vi "MasterAquisitionFile_LD_IOS.vi"() -> ()   [LabVIEW 2018]
uses:
  <vilib>/userdefined/High Color/IMAQdx.ctl
  <vilib>/vision/driver/IMAQdx.llb/IMAQdx Camera Control Mode.ctl
  <vilib>/vision/driver/IMAQdx.llb/IMAQdx Acquisition Mode.ctl
  <vilib>/vision/driver/IMAQdx.llb/IMAQdx Buffer Number Mode.ctl
  <vilib>/DAQmx/write.llb/DAQmx Write (Digital Bool 1Line 1Point).vi
  <vilib>/DAQmx/read.llb/DAQmx Read (Analog 1D Wfm NChan NSamp).vi
  <vilib>/DAQmx/write.llb/DAQmx Write (Digital 1D Bool NChan 1Samp 1Line).vi
  <vilib>/DAQmx/create/channels.llb/DAQmx Create Channel (DO-Digital Output).vi
  <vilib>/DAQmx/create/channels.llb/DAQmx Create Channel (CO-Pulse Generation-Frequency).vi
  <vilib>/DAQmx/configure/timing.llb/DAQmx Timing (Implicit).vi
  <vilib>/DAQmx/create/channels.llb/DAQmx Create Channel (AI-Voltage-Basic).vi
  <vilib>/DAQmx/configure/timing.llb/DAQmx Timing (Sample Clock).vi
  <vilib>/DAQmx/configure/trigger.llb/DAQmx Start Trigger (Digital Edge).vi
  <vilib>/DAQmx/miscellaneous.llb/DAQmx Fill In Error Info.vi
  <vilib>/vision/driver/NI_Vision_Acquisition_Software.lvlib
  <resource>/objmgr/imaqdx.rc
panel:
  out "Dev2 Analog Samples":i32
  out "Dev2 Analog":bool
  in  "stop 2":bool
  out "CBV Camera 2":bool
  in  "Dev2 Channels":tag="Dev2/ai4:5"
  in  "Dev2 Analog Channels":string[](array[string])=["LD_BackScatter", "LD_Flow", "LPadSol", "RPadSol", "AudSol", "Hippocampus", "EMG", "Cortical_RH"]
  out "?":T1(plugin-control)
  out "?":T1(plugin-control)
  out "?":T1(plugin-control)
  out "?":T1(plugin-control)
  in  "stop":bool
  out "CBV Cam":bool
  out "Pupil Cam":bool
  out "Whisk Cam":bool
  out "Web Cam":bool
  out "Dev1 Analog":bool
  in  "Dev1 Channels":tag="Dev1/ai0:7"
  out "Web Cam Fs":dbl(knob) scale=0.0..200.0
  out "CBV Cam":dbl(knob) scale=0.0..200.0
  out "Whisk Cam Fs":dbl(knob) scale=0.0..200.0
  out "Last Whisk\nBuffer 2":u32
  out "Pupil Cam Fs":dbl(knob) scale=0.0..200.0
  out "Dropped 2":u32(slide) caption="Pupil Cam" scale=0.0..90.0
  in  "Pupil Cam ID":T2="cam2"
  in  "Pupil Cam Trig Source":tag="Dev2/ctr0"
  in  "Exposure Time (microsec)":string="10000"
  out "Solenoids":bool[](array[boolean])
  out "Dev1 Analog Samples":i32
  in  "Dev1 Analog Channels":string[](array[string])=["Cortical_LH", "Force_Sensor", "LPadSol", "RPadSol", "AudSol", "Hippocampus", "EMG", "Cortical_RH"]
  in  "Whisker Cam ID":T2="cam1"
  in  "WebCam ID":T2="cam0"
  in  "Analog Acquisition":cluster{"Analog Fs":u16}={"Analog Fs"=20000} {"Analog Fs" format="%0.0f"}
  in  "Camera Acquisition Setup":T3={"CBV Cam Fs"=30, "Whisk Cam Fs"=150, "Web Cam Fs"=15, "Pupil Cam Fs"=30}
  out "Notes Size":i32=7
  out "Notes Reversed":string[](array[string])=["Experimenter", "Animal ID", "Hemisphere", "Solenoid PSI", "Isoflurane time", "Session ID", "Amplifier Gain"]
  out "Notes Array":string[](array[string])=["Amplifier Gain", "Session ID", "Isoflurane time", "Solenoid PSI", "Hemisphere", "Animal ID", "Experimenter"]
  in  "Notes:":T4={"Experimenter"="Kevin", "Animal ID"="T109", "Hemisphere"="Both", "Solenoid PSI"="10", "Isoflurane time"="1320", "Session ID"="Imaging Session Seven", "Amplifier Gain"="10000"}
  in  "Whisk Cam Trig Source":tag="Dev1/ctr1"
  in  "CBV Cam Trig Source":tag="Dev1/ctr0"
  in  "Left Pad":tag="Dev1/port0/line0"
  in  "Right Pad":tag="Dev1/port0/line1"
  in  "Auditory":tag="Dev1/port0/line2"
  in  "Offset (s)":dbl=15.0
  in  "Duration (s)":dbl=0.1 step=0.1
  in  "Interval (s)":dbl=30.0
  in  "Right Pad":dbl=1.0
  in  "Left Pad":dbl=1.0
  in  "Auditory":dbl=1.0
  in  "Target Path":path=path "D:/T109/Imaging Session Seven 9.5.19" caption="Final saved file location"
  out "Dropped":u32(slide) caption="Whisk Cam" scale=0.0..450.0
  out "Current file name":string="190905_13_40_55"
  out "CBV Camera":bool
  out "Time Elapsed (Min)":cluster{dbl, dbl}(slide)={15.0, 0.00046676000000000004} scale=0.0..15.0 scale format="%#_2g"
  in  "Time (min)":dbl(knob)=15.0 min=0.5 max=20.0 step=0.5 scale=0.0..20.0 scale format="%#_2g"
  in  "Temp Path":path=path "D:/LabVIEW Streamed Data" caption="Temporary path for streamed data"
  out "Last CBV\nBuffer":i32
  out "Last Whisk\nBuffer":u32=5
  # "Stimuli"
  # "LPAD"
  # "RPAD"
  # "AUD"
  # "Whisk Cam ID"
  # "Pupil Cam ID"
  # "Ratio"
  # "Web Cam ID"
  # "Data Sampling Rates"
  # "Ratio"
  # "Ratio"
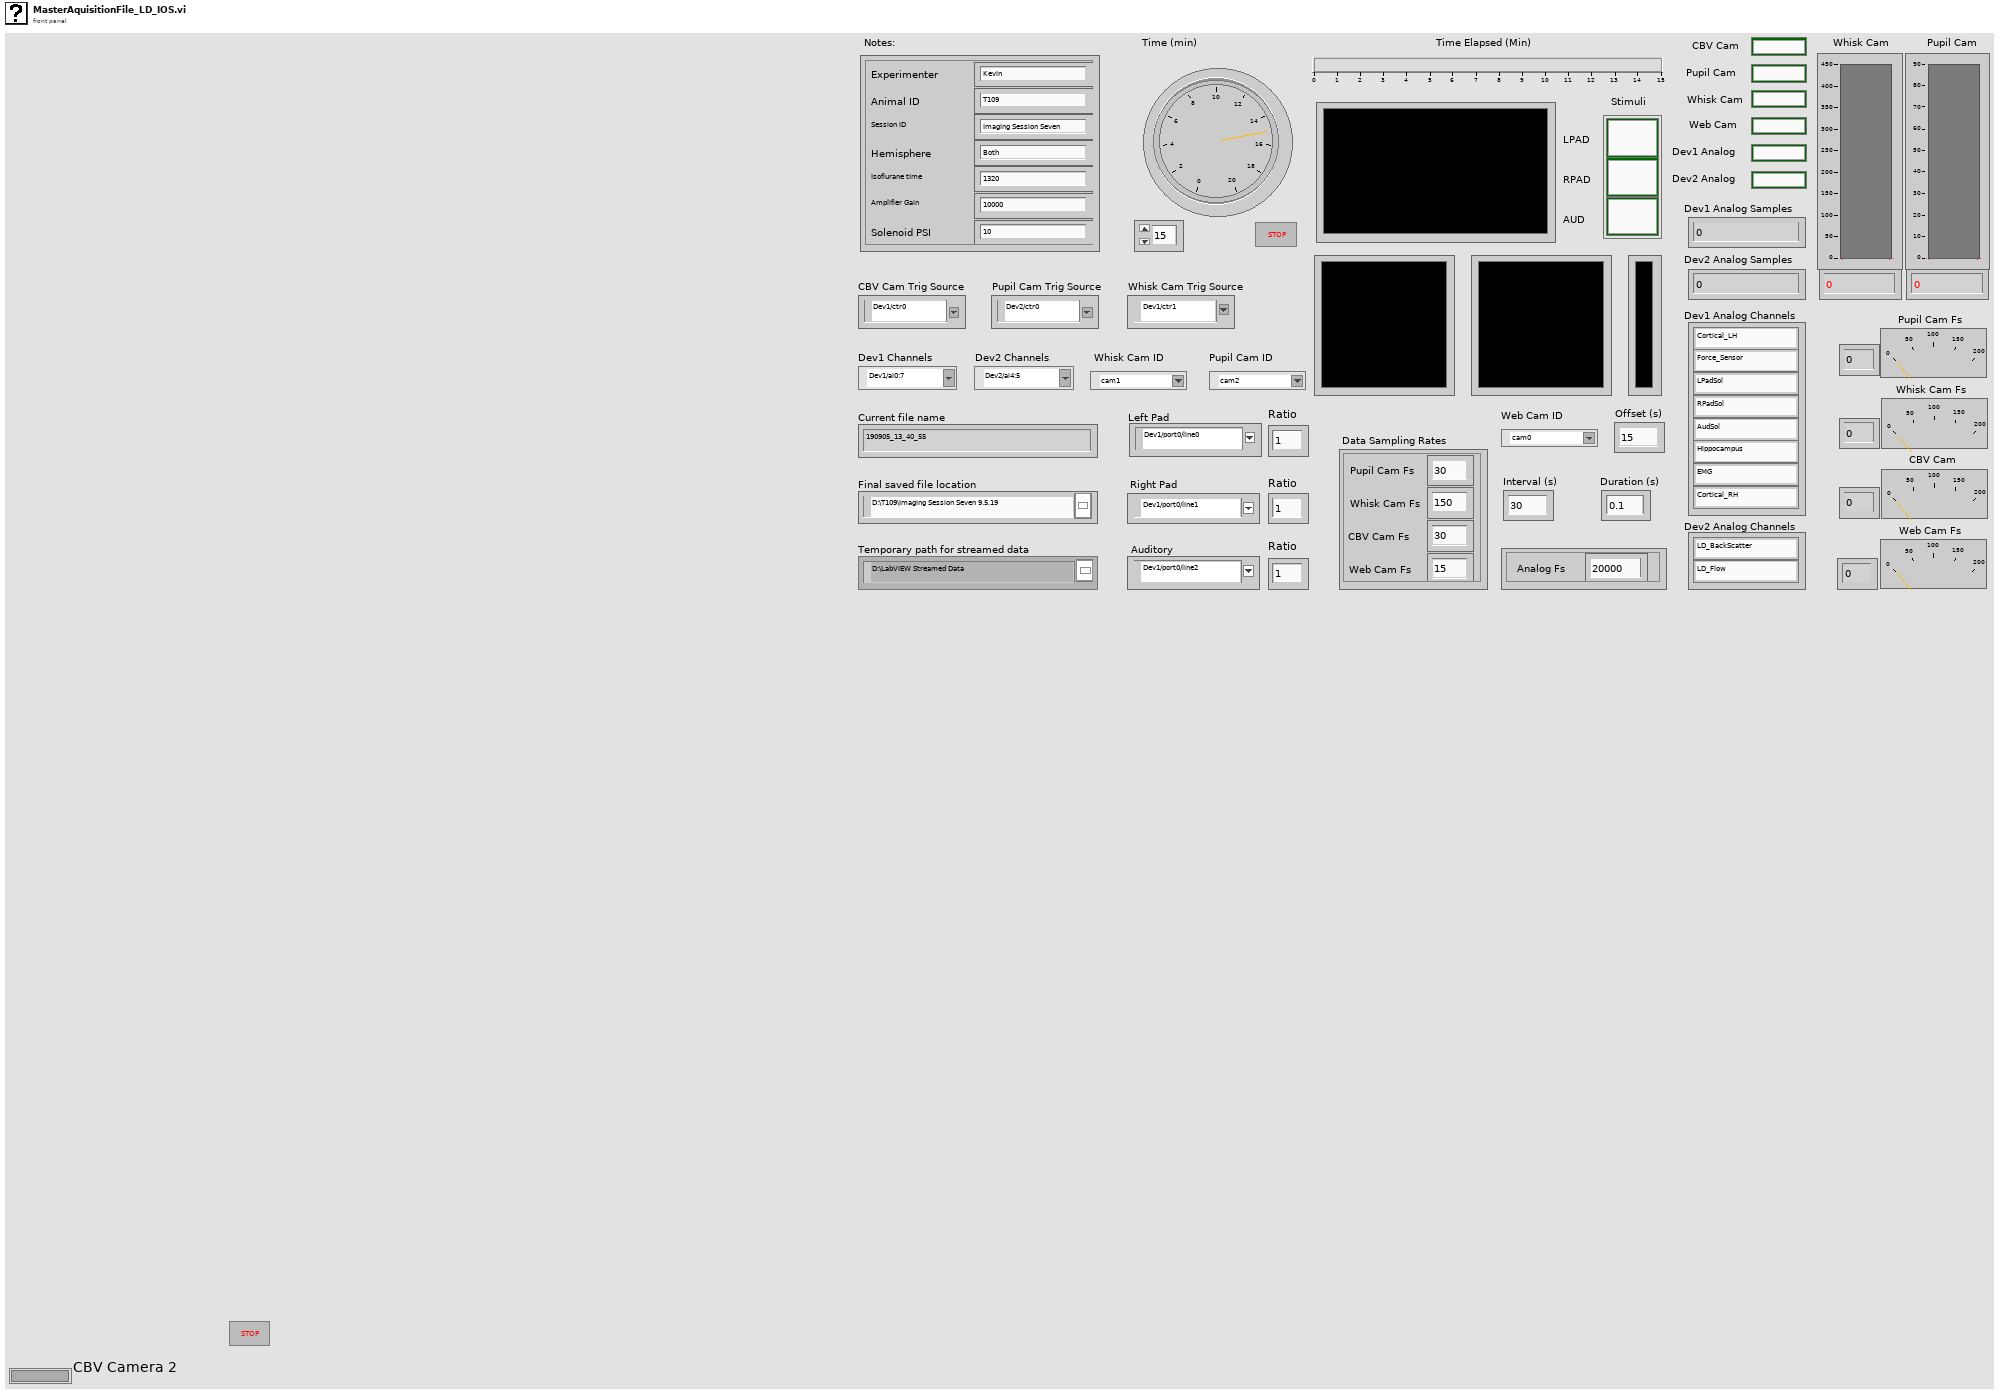
[diagram p1: front panel]
types:
  T1 = typedef "IMAQ Image.ctl" = refnum<image>
  T2 = typedef "IMAQdx.ctl" = refnum<k21>
  T3 = cluster{"CBV Cam Fs":u16, "Whisk Cam Fs":u16, "Web Cam Fs":u16, "Pupil Cam Fs":u16}
  T4 = cluster{"Experimenter":string, "Animal ID":string, "Hemisphere":string, "Solenoid PSI":string, "Isoflurane time":string, "Session ID":string, "Amplifier Gain":string}
  T5 = enum16{"open", "open or create", "create or replace", "create", "open (read-only)"}
  T6 = enum16{"open", "replace", "create", "open or create", "replace or create", "replace or create with confirmation"}
  T7 = typedef "Image Type" = u32
  T8 = typedef "NI_Vision_Acquisition_Software.lvlib/IMAQdx Acquisition Mode.ctl" = enum32{"One Shot", "Continuous"}
  T9 = typedef "NI_Vision_Acquisition_Software.lvlib/IMAQdx Camera Control Mode.ctl" = enum32{"Controller", "Listener"}
  T10 = typedef "IMAQ AVI2 Refnum.ctl" = refnum<k20>
  T11 = enum16{"big-endian, network order", "native, host order", "little-endian"}
  T12 = typedef "NI_Vision_Acquisition_Software.lvlib/IMAQdx Buffer Number Mode.ctl" = enum32{"Next", "Last", "Buffer Number", "Every", "Last New"}
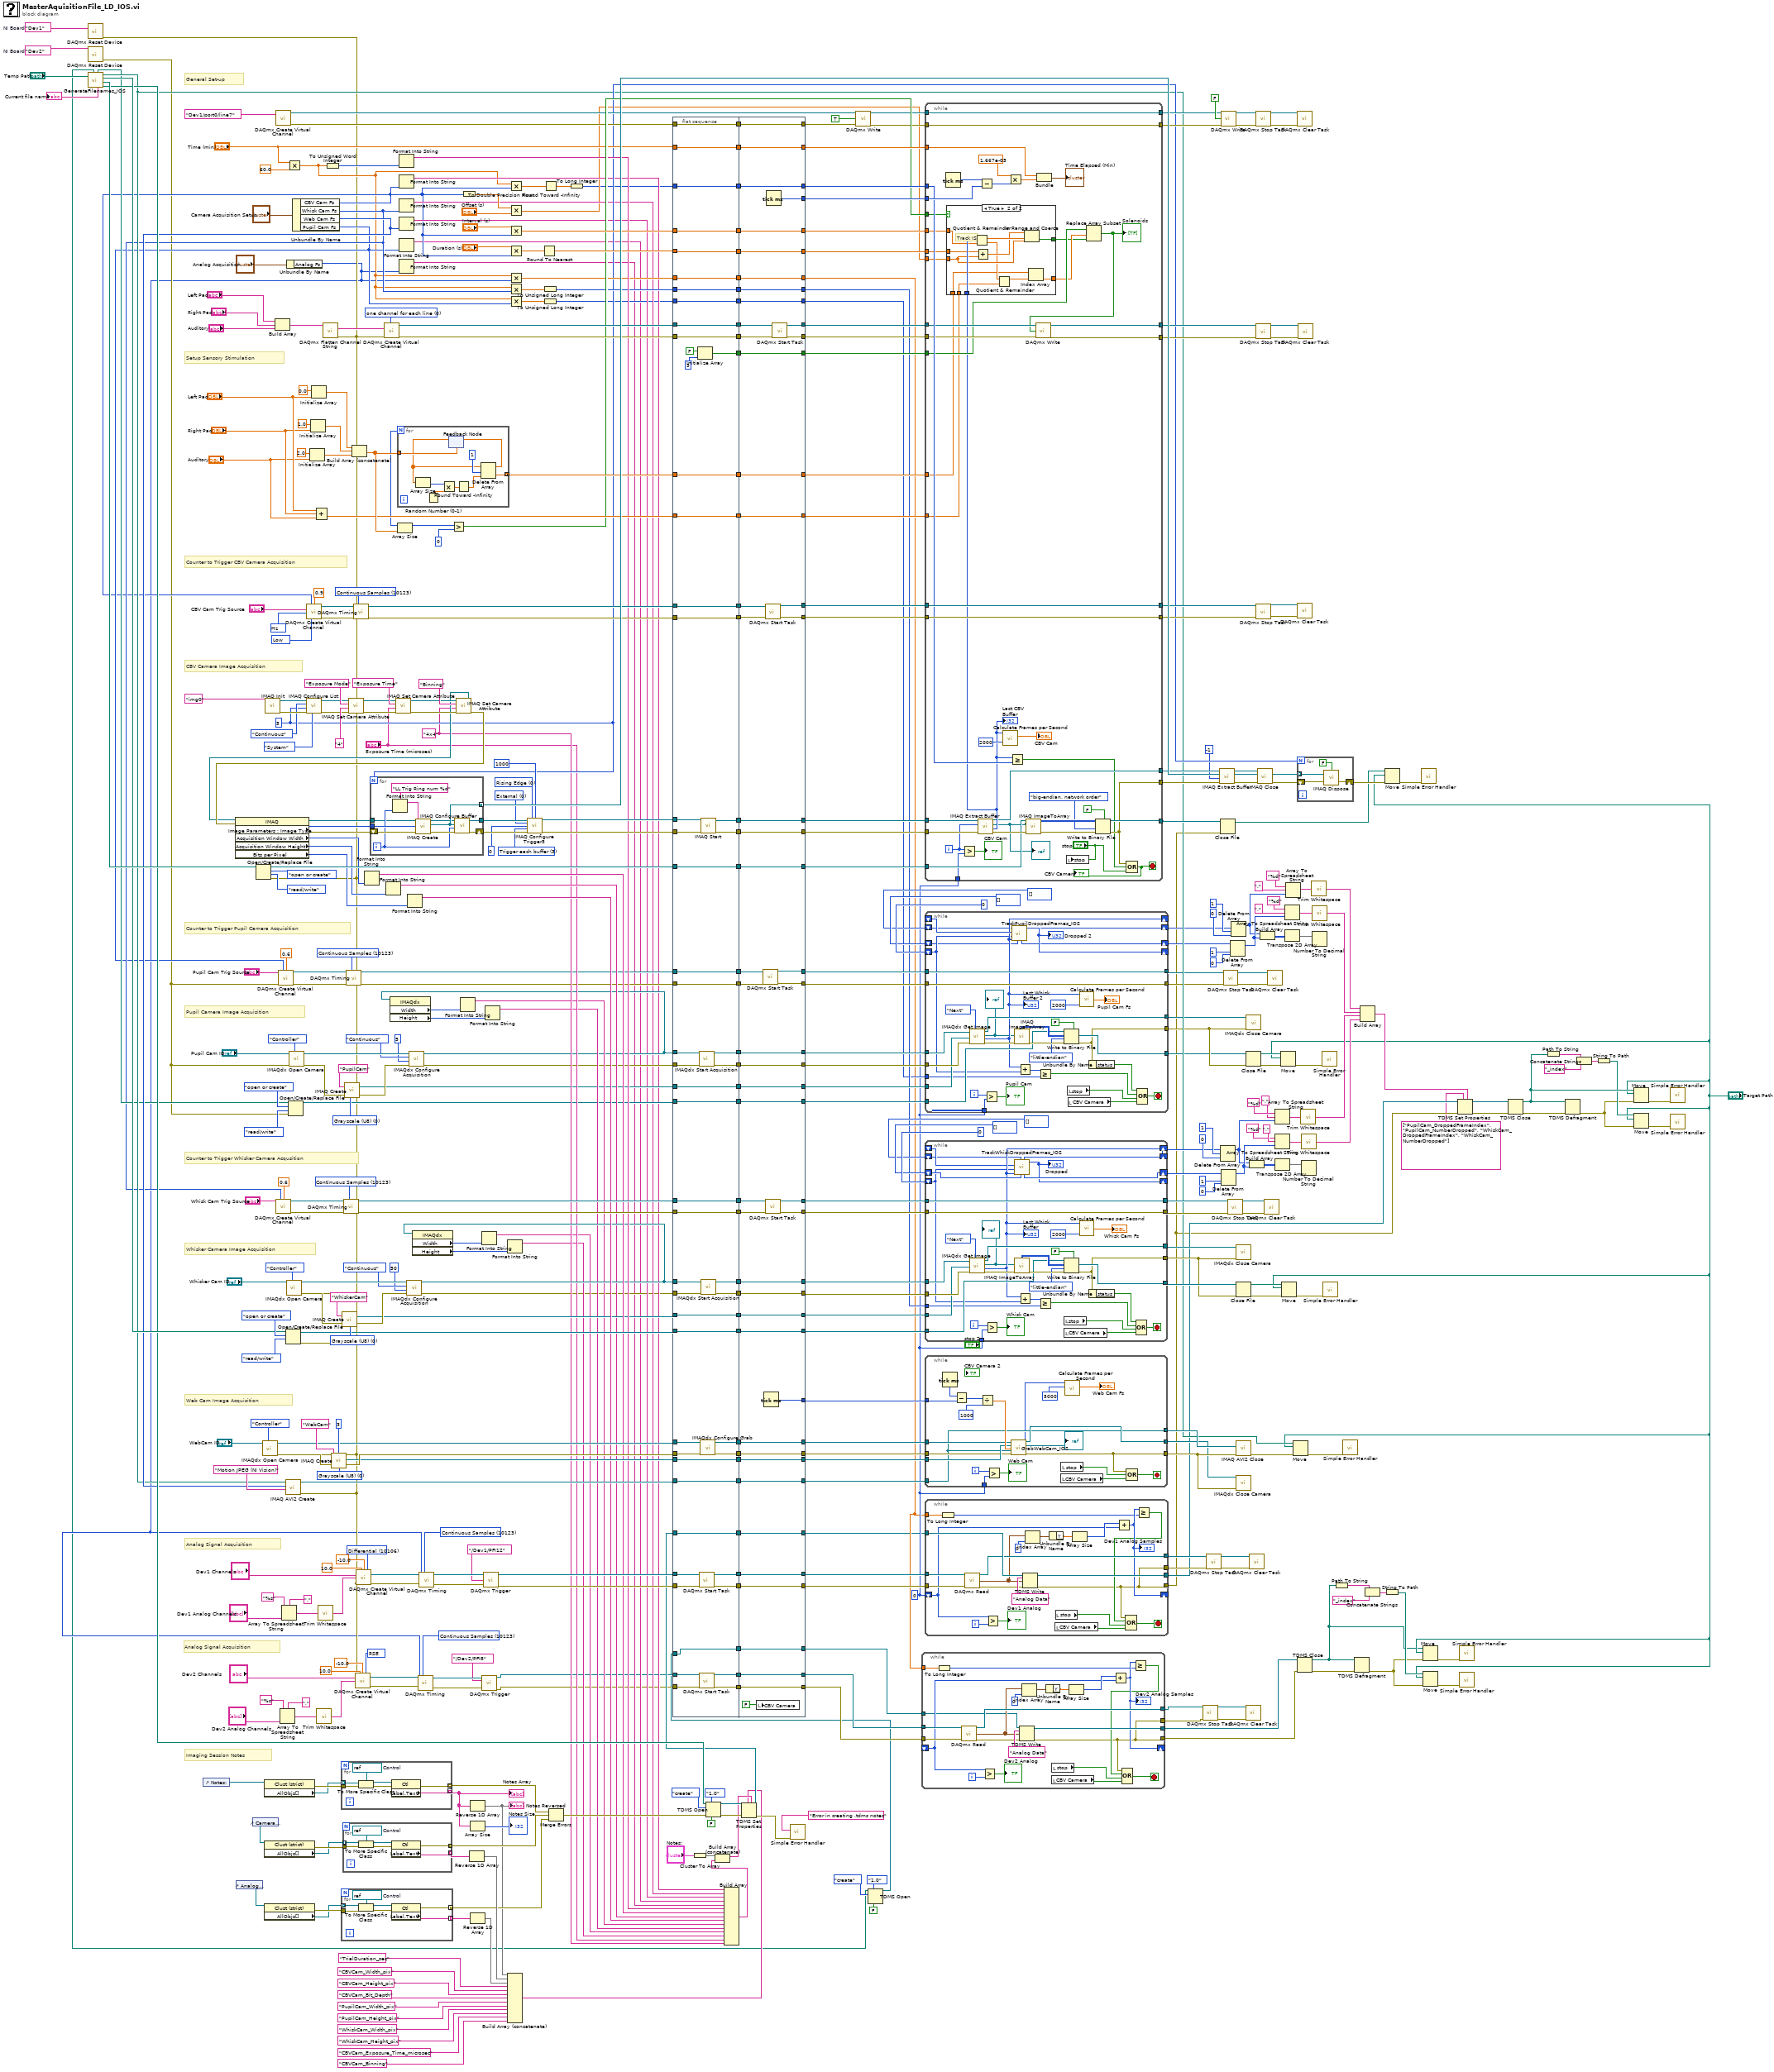
[diagram p0: block diagram]
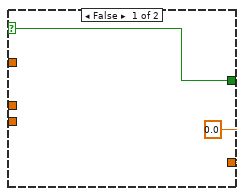
[diagram p2: hidden frame]
diagram:
  w46 = 10123 items=["Finite Samples"=10178, "Continuous Samples"=10123, "Hardware Timed Single Point"=12522] ("sample mode")
  w49 = 10083 items=["default"=-1, "RSE"=10083, "NRSE"=10078, "Differential"=10106, "Pseudodifferential"=12529] ("input terminal configuration")
  w66 = tag "Dev2"  # NI Board
  w153 = 10123 items=["Finite Samples"=10178, "Continuous Samples"=10123, "Hardware Timed Single Point"=12522] ("sample mode")
  w160 = T7 0 items=["Grayscale (U8)", "Grayscale (I16)", "Grayscale (SGL)", "Complex (CSG)", "RGB (U32)", "HSL (U32)", "RGB (U64)", "Grayscale (U16)"] ("Image Type")
  w142 = "4x4" ("Attribute Value")
  w72 = 0
  w326 = 0 items=["one channel for each line", "one channel for all lines"] ("line grouping")
  w377 = 10123 items=["Finite Samples"=10178, "Continuous Samples"=10123, "Hardware Timed Single Point"=12522] ("sample mode")
  w380 = 10106 items=["default"=-1, "RSE"=10083, "NRSE"=10078, "Differential"=10106, "Pseudodifferential"=12529] ("input terminal configuration")
  w431 = T7 0 items=["Grayscale (U8)", "Grayscale (I16)", "Grayscale (SGL)", "Complex (CSG)", "RGB (U32)", "HSL (U32)", "RGB (U64)", "Grayscale (U16)"] ("Image Type")
  w451 = u32 0 items=["Rising Edge", "Falling Edge"] ("Trigger Polarity")
  w454 = u32 0 items=["External"=0, "RTSI"=1, "ISO In"=2, "Scaled Encoder"=5] ("Trigger Type")
  w445 = tag "Dev1"  # NI Board
  w446 = 10123 items=["Finite Samples"=10178, "Continuous Samples"=10123, "Hardware Timed Single Point"=12522] ("sample mode")
  w449 = 10373 items=["Hz"=10373] ("units")
  w450 = 10214 items=["High"=10192, "Low"=10214] ("idle state")
  w172 = u32 5 ("Number of Buffers")
  w452 = u32 3 items=["Disabled", "Trigger start of acquisition", "Trigger start of each buffer list", "Trigger each buffer", "Trigger each line (linescan)", "Trigger end of acquisition"] ("Action")
  w466 = 10123 items=["Finite Samples"=10178, "Continuous Samples"=10123, "Hardware Timed Single Point"=12522] ("sample mode")
  w473 = T7 0 items=["Grayscale (U8)", "Grayscale (I16)", "Grayscale (SGL)", "Complex (CSG)", "RGB (U32)", "HSL (U32)", "RGB (U64)", "Grayscale (U16)"] ("Image Type")
  # "Analog Signal Acquisition"
  # "General Set-up"
  # "Pupil Camera Image Acquisition"
  # "Counter to Trigger Pupil Camera Acquisition"
  # "Whisker Camera Image Acquisition"
  # "Imaging Session Notes"
  # "Setup Sensory Stimulation"
  # "CBV Camera Image Acquisition"
  # "Counter to Trigger CBV Camera Acquisition"
  # "Counter to Trigger Whisker Camera Acqusition"
  # "Web Cam Image Acquisition"
  # "Analog Signal Acquisition"
  n1 = call <vilib>:"DAQmx Reset Device.vi"("device in"=w445) -> ("error out"=w35:errorcluster)  [unwired: 14 in]
  n2 = call <vilib>:"DAQmx Reset Device.vi"("device in"=w66) -> ("error out"=w65:errorcluster)  [unwired: 14 in]
  n3 = call "GenerateFilenames_IOS.vi"("path"="Temp Path") -> ("TDMS Path"=w282:path, "Dalsa Path"=w438:path, "Basler Path"=w434:path, "WebCam Path"=w171:path, "Analog file name"=→"Current file name":string, "Basler2 Path"=w151:path, "TDMS Path 2"=w2:path)  [unwired: 3 in, 1 out]
  n4 = control-ref of="Notes:"() -> (w287:refnum<vi>)
  n5 = control-ref of="Analog Acquisition"() -> (w265:refnum<vi>)
  n6 = control-ref of="Camera Acquisition Setup"() -> (w266:refnum<vi>)
  n7 = Open/Create/Replace File(file path (use dialog)=w438, error in=w35, operation (0:open)=T6."open or create", access (0:read/write)=enum16{"read/write", "read-only", "write-only"}."read/write") -> (refnum out=w381:refnum<file>)  [unwired: 2 in, 2 out]
  n8 = call <vilib>:"IMAQdx Open Camera.vi"("Camera Control Mode"=IMAQdx_Camera_Control_Mode."Controller", "error in"=w35, "Session In"="WebCam ID") -> ("error out"=w427:errorcluster, "Session Out"=w425:T2)  [unwired: 7 in]
  n9 = property class="Clust (strict)"(reference=w287) -> (error out=w290:errorcluster, "AllObjs[]"=w179:refnum<vi>[])  [unwired: 1 in, 1 out]
  n10 = property class="Clust (strict)"(reference=w266) -> (error out=w285:errorcluster, "AllObjs[]"=w180:refnum<vi>[])  [unwired: 1 in, 1 out]
  n11 = property class="Clust (strict)"(reference=w265) -> (error out=w264:errorcluster, "AllObjs[]"=w178:refnum<vi>[])  [unwired: 1 in, 1 out]
  n12 = call <vilib>:"IMAQ Init.vi"("error in (no error)"=w35, "Interface Name"="img0") -> ("error out"=w464:errorcluster, "IMAQ Session Out"=w465:refnum<k11>)  [unwired: 8 out]
  n13 = Build Array("Left Pad", "Right Pad", "Auditory") -> (w58:tag[])
  n14 = call-poly <vilib>:"DAQmx Create Virtual Channel.vi"("lines"=tag "Dev1/port0/line7") -> ("task out"=w212:refnum<k21>, "error out"=w215:errorcluster)  [unwired: 13 in]
  n15 = Array To Spreadsheet String(delimiter (Tab)=",", array="Dev2 Analog Channels", 3:"%s" ("format string")) -> (spreadsheet string=w39:string)
  n16 = Array To Spreadsheet String(delimiter (Tab)=",", array="Dev1 Analog Channels", 3:"%s" ("format string")) -> (spreadsheet string=w251:string)
  n17 = Open/Create/Replace File(file path (use dialog)=w434, error in=w35, operation (0:open)=T6."open or create", access (0:read/write)=enum16{"read/write", "read-only", "write-only"}."read/write") -> (refnum out=w399:refnum<file>)  [unwired: 2 in, 2 out]
  n18 = Unbundle By Name("Analog Acquisition") -> ("Analog Fs"=w34:u16)
  n19 = call <vilib>:"IMAQdx Open Camera.vi"("Camera Control Mode"=IMAQdx_Camera_Control_Mode."Controller", "error in"=w35, "Session In"="Whisker Cam ID") -> ("error out"=w476:errorcluster, "Session Out"=w479:T2)  [unwired: 7 in]
  n20 = Multiply(x="Time (min)", y=60.0) -> (x*y=w74:dbl)
  n21 = Open/Create/Replace File(file path (use dialog)=w151, error in=w65, operation (0:open)=T6."open or create", access (0:read/write)=enum16{"read/write", "read-only", "write-only"}."read/write") -> (refnum out=w132:refnum<file>)  [unwired: 2 in, 2 out]
  n22 = call <vilib>:"IMAQdx Open Camera.vi"("Camera Control Mode"=IMAQdx_Camera_Control_Mode."Controller", "error in"=w65, "Session In"="Pupil Cam ID") -> ("error out"=w163:errorcluster, "Session Out"=w166:T2)  [unwired: 7 in]
  n23 = Unbundle By Name("Camera Acquisition Setup") -> ("CBV Cam Fs"=w76:u16, "Whisk Cam Fs"=w114:u16, "Web Cam Fs"=w259:u16, "Pupil Cam Fs"=w108:u16)
  n24 = call-poly <vilib>:"DAQmx Create Virtual Channel.vi"("frequency"=w114, "duty cycle"=0.6, "counter"="Whisk Cam Trig Source", "error in"=w35) -> ("task out"=w468:refnum<k21>, "error out"=w467:errorcluster)  [unwired: 10 in]
  n25 = call-poly <vilib>:"DAQmx Create Virtual Channel.vi"("frequency"=w108, "duty cycle"=0.6, "counter"="Pupil Cam Trig Source", "error in"=w65) -> ("task out"=w155:refnum<k21>, "error out"=w154:errorcluster)  [unwired: 10 in]
  n26 = call "IMAQ AVI2 Create"("error in (no error)"=w35, "Codec"="Motion JPEG (NI Vision)", "Frames Per Second"=w259, "AVI Path"=w171) -> ("AVI Refnum"=w417:T10)  [unwired: 6 in, 1 out]
  n27 = call <vilib>:"IMAQ Configure List.vi"("Memory Location"=enum16{"System", "Onboard"}."System", "error in (no error)"=w464, "Number of buffers"=w172, "Continuous?"=enum16{"One-Shot", "Continuous"}."Continuous" ("Continuous ?"), "IMAQ Session In"=w465) -> ("error out"=w193:errorcluster, "IMAQ Session Out"=w189:refnum<k11>)  [unwired: 1 in, 4 out]
  n28 = call-poly <vilib>:"DAQmx Create Virtual Channel.vi"("frequency"=w76, "duty cycle"=0.9, "counter"="CBV Cam Trig Source", "units"=w449, "error in"=w35, "idle state"=w450) -> ("task out"=w448:refnum<k21>, "error out"=w447:errorcluster)  [unwired: 8 in]
  n29 = Initialize Array(2.0 ("element"), "Auditory") -> (w70:dbl[])
  n30 = Initialize Array(1.0 ("element"), "Right Pad") -> (w330:dbl[])
  n31 = Initialize Array(0.0 ("element"), "Left Pad") -> (w331:dbl[])
  n32 = Compound Arithmetic op=ADD("Left Pad", "Right Pad", "Auditory") -> (w310:dbl)
  n33 = call <vilib>:"Trim Whitespace.vi"("string"=w39) -> ("trimmed string"=w38:string)  [unwired: 1 in]
  n34 = call <vilib>:"Trim Whitespace.vi"("string"=w251) -> ("trimmed string"=w250:string)  [unwired: 1 in]
  n35 = call <vilib>:"DAQmx Flatten Channel String.vi"("names in"=w58, "error in"=w35) -> ("names out"=w292:string, "error out"=w291:errorcluster)  [unwired: 12 in]
  n36 = To Unsigned Word Integer(number=w74) -> (unsigned 16bit integer=w245:u16)
  n37 = call "IMAQ Create"("Border Size"=3, "Image Name"="WebCam", "Image Type"=w431, "error in (no error)"=w427) -> ("New Image"=w424:T1, "error out"=w426:errorcluster)  [unwired: 1 in]
  n38 = for {
    tunnel: [w485] -> w289 mode=indexing
    tunnel: w290 -> [w484]
    tunnel: [w482] -> w273 mode=indexing
    tunnel: w179 -> [w481] mode=indexing
    w486 = refnum<vi> refnum  # Control
    n39 = To More Specific Class(target class=w486, reference=w481, error in=w484) -> (specific class reference=w487:refnum<vi>, error out=w483:errorcluster)
    n40 = property class="Ctl"(reference=w487, error in=w483) -> (error out=w482:errorcluster, "Label.Text"=w485:string)  [unwired: 1 out]
  }
  "Notes Array" <- w289
  n41 = for {
    tunnel: [w492] -> w262 mode=indexing
    tunnel: w264 -> [w491]
    tunnel: [w489] -> w263 mode=indexing
    tunnel: w178 -> [w488] mode=indexing
    w493 = refnum<vi> refnum  # Control
    n42 = To More Specific Class(target class=w493, reference=w488, error in=w491) -> (specific class reference=w494:refnum<vi>, error out=w490:errorcluster)
    n43 = property class="Ctl"(reference=w494, error in=w490) -> (error out=w489:errorcluster, "Label.Text"=w492:string)  [unwired: 1 out]
  }
  n44 = call "IMAQ Create"("Image Name"="WhiskerCam", "Image Type"=w473, "error in (no error)"=w476) -> ("New Image"=w232:T1, "error out"=w474:errorcluster)  [unwired: 2 in]
  n45 = for {
    tunnel: [w499] -> w286 mode=indexing
    tunnel: w285 -> [w498]
    tunnel: [w496] -> w272 mode=indexing
    tunnel: w180 -> [w495] mode=indexing
    w500 = refnum<vi> refnum  # Control
    n46 = To More Specific Class(target class=w500, reference=w495, error in=w498) -> (specific class reference=w501:refnum<vi>, error out=w497:errorcluster)
    n47 = property class="Ctl"(reference=w501, error in=w497) -> (error out=w496:errorcluster, "Label.Text"=w499:string)  [unwired: 1 out]
  }
  n48 = call-poly <vilib>:"DAQmx Timing.vi"("task/channels in"=w468, "sample mode"=w466, "error in"=w467) -> ("task out"=w362:refnum<k21>, "error out"=w360:errorcluster)  [unwired: 11 in]
  n49 = call "IMAQ Create"("Image Name"="PupilCam", "Image Type"=w160, "error in (no error)"=w163) -> ("New Image"=w117:T1, "error out"=w161:errorcluster)  [unwired: 2 in]
  n50 = call-poly <vilib>:"DAQmx Timing.vi"("task/channels in"=w155, "sample mode"=w153, "error in"=w154) -> ("task out"=w130:refnum<k21>, "error out"=w128:errorcluster)  [unwired: 11 in]
  n51 = call <vilib>:"IMAQ Set Camera Attribute.vi"("error in (no error)"=w193, "Attribute Value"="4", "Camera Attribute"="Exposure Mode", "IMAQ Session In"=w189) -> ("error out"=w192:errorcluster, "IMAQ Session Out"=w188:refnum<k11>)  [unwired: 4 in]
  n52 = Build Array (concatenate)(w331, w330, w70) -> (w329:dbl[])
  n53 = call-poly <vilib>:"DAQmx Timing.vi"("task/channels in"=w448, "sample mode"=w446, "error in"=w447) -> ("task out"=w366:refnum<k21>, "error out"=w364:errorcluster)  [unwired: 11 in]
  n54 = call-poly <vilib>:"DAQmx Create Virtual Channel.vi"("maximum value"=10.0, "minimum value"=-10.0, "input terminal configuration"=w49, "physical channels"="Dev2 Channels", "name to assign"=w38, "error in"=w35) -> ("task out"=w48:refnum<k21>, "error out"=w47:errorcluster)  [unwired: 8 in]
  n55 = call-poly <vilib>:"DAQmx Create Virtual Channel.vi"("maximum value"=10.0, "minimum value"=-10.0, "input terminal configuration"=w380, "physical channels"="Dev1 Channels", "name to assign"=w250, "error in"=w35) -> ("task out"=w379:refnum<k21>, "error out"=w378:errorcluster)  [unwired: 8 in]
  n56 = call-poly <vilib>:"DAQmx Create Virtual Channel.vi"("lines"=w292, "line grouping"=w326, "error in"=w291) -> ("task out"=w324:refnum<k21>, "error out"=w322:errorcluster)  [unwired: 11 in]
  n57 = call <vilib>:"IMAQ Set Camera Attribute.vi"("error in (no error)"=w192, "Attribute Value"="Exposure Time (microsec)", "Camera Attribute"="Exposure Time", "IMAQ Session In"=w188) -> ("error out"=w191:errorcluster, "IMAQ Session Out"=w187:refnum<k11>)  [unwired: 4 in]
  n58 = Array Size(array=w329) -> (size(s)=w256:i32)
  n59 = for {
    N: w256 -> [_]
    tunnel: w329 -> [w505]
    tunnel: [w502] -> w307 mode=concatenating
    n60 = Random Number (0-1)() -> (number: 0 to 1=w509:dbl)
    n61 = feedback #1(w505) -> (w504:dbl[])
    n62 = Array Size(array=w504) -> (size(s)=w510:i32)
    n63 = Multiply(x=w510, y=w509) -> (x*y=w508:dbl)
    n64 = Round Toward -Infinity(1:w508) -> (0:w507:dbl)
    n65 = Delete From Array(array=w504, length=1, index=w507) -> (deleted portion=w502:dbl[], array with subset deleted=w503:dbl[])
    n66 = feedback-in #1(w503) -> ()
  }
  n67 = Format Into String(w245) -> (resulting string=w247:string)  [unwired: 3 in, 1 out]
  n68 = Format Into String(w76) -> (resulting string=w112:string)  [unwired: 3 in, 1 out]
  n69 = Format Into String(w114) -> (resulting string=w111:string)  [unwired: 3 in, 1 out]
  n70 = Format Into String(w259) -> (resulting string=w110:string)  [unwired: 3 in, 1 out]
  n71 = Format Into String(w108) -> (resulting string=w51:string)  [unwired: 3 in, 1 out]
  n72 = Format Into String(w34) -> (resulting string=w50:string)  [unwired: 3 in, 1 out]
  n73 = call <vilib>:"IMAQdx Configure Acquisition.vi"("error in"=w474, "Number of Buffers"=u32 50, "Continuous?"=IMAQdx_Acquisition_Mode."Continuous", "Session In"=w479) -> ("error out"=w73:errorcluster, "Session Out"=w233:T2)  [unwired: 6 in]
  n74 = call <vilib>:"IMAQdx Configure Acquisition.vi"("error in"=w161, "Number of Buffers"=u32 5, "Continuous?"=IMAQdx_Acquisition_Mode."Continuous", "Session In"=w166) -> ("error out"=w134:errorcluster, "Session Out"=w118:T2)  [unwired: 6 in]
  n75 = property class="IMAQdx"(reference=w118) -> ("Width"=w150:u32, "Height"=w149:u32)  [unwired: 1 in, 2 out]
  n76 = property class="IMAQdx"(reference=w233) -> ("Width"=w244:u32, "Height"=w243:u32)  [unwired: 1 in, 2 out]
  n77 = call-poly <vilib>:"DAQmx Timing.vi"("task/channels in"=w48, "sample mode"=w46, "rate"=w34, "error in"=w47) -> ("task out"=w36:refnum<k21>, "error out"=w45:errorcluster)  [unwired: 10 in]
  n78 = call-poly <vilib>:"DAQmx Timing.vi"("task/channels in"=w379, "sample mode"=w377, "rate"=w34, "error in"=w378) -> ("task out"=w176:refnum<k21>, "error out"=w376:errorcluster)  [unwired: 10 in]
  n79 = Greater?(x=w256, y=0) -> (0:w254:bool)
  n80 = call <vilib>:"IMAQ Set Camera Attribute.vi"("error in (no error)"=w191, "Attribute Value"=w142, "Camera Attribute"="Binning", "IMAQ Session In"=w187) -> ("error out"=w190:errorcluster, "IMAQ Session Out"=w186:refnum<k11>)  [unwired: 4 in]
  n81 = property class="IMAQ"(reference=w186, error in=w190) -> (reference out=w200:refnum<k11>, error out=w199:errorcluster, "Image Parameters : Image Type"=w460:u32, "Acquisition Window Width"=w242:u32, "Acquisition Window Height"=w241:u32, "Bits per Pixel"=w240:u32)
  n82 = Format Into String(w242) -> (resulting string=w239:string)  [unwired: 3 in, 1 out]
  n83 = for {
    N: w172 -> [_]
    tunnel: [w520] -> w456
    tunnel: w460 -> [w518]
    shift-right: [w519] -> w455
    shift-left: w199 -> [w517]
    tunnel: [w512] -> w457 mode=indexing
    tunnel: w200 -> [w511]
    i -> [w513]
    n84 = Format Into String(format string="LL Trig Ring num %d", w513) -> (resulting string=w515:string)  [unwired: 2 in, 1 out]
    n85 = call "IMAQ Create"("Image Name"=w515, "Image Type"=w518, "error in (no error)"=w517) -> ("New Image"=w512:T1, "error out"=w516:errorcluster)  [unwired: 1 in, 1 out]
    n86 = call <vilib>:"IMAQ Configure Buffer.vi"("error in (no error)"=w516, "Buffer Number"=w513, "Image In"=w512, "IMAQ Session In"=w511) -> ("error out"=w519:errorcluster, "IMAQ Session Out"=w520:refnum<k11>)  [unwired: 2 in, 4 out]
  }
  n87 = Format Into String(w241) -> (resulting string=w173:string)  [unwired: 3 in, 1 out]
  n88 = Format Into String(w240) -> (resulting string=w238:string)  [unwired: 3 in, 1 out]
  n89 = Format Into String(w150) -> (resulting string=w137:string)  [unwired: 3 in, 1 out]
  n90 = To Double Precision Float(number=w76) -> (double precision float=w293:dbl)
  n91 = Reverse 1D Array(array=w286) -> (reversed array=w276:string[])
  n92 = Reverse 1D Array(array=w289) -> (reversed array=w177:string[])
  "Notes Reversed" <- w177
  n93 = Array Size(array=w289) -> (size(s)=→"Notes Size":i32)
  n94 = Reverse 1D Array(array=w262) -> (reversed array=w261:string[])
  n95 = Format Into String(w244) -> (resulting string=w139:string)  [unwired: 3 in, 1 out]
  n96 = call-poly <vilib>:"DAQmx Trigger.vi"("task/channels in"=w36, "source"=tag "/Dev2/PFI8", "error in"=w45) -> ("task out"=w33:refnum<k21>, "error out"=w32:errorcluster)  [unwired: 11 in]
  n97 = call-poly <vilib>:"DAQmx Trigger.vi"("task/channels in"=w176, "source"=tag "/Dev1/PFI12", "error in"=w376) -> ("task out"=w375:refnum<k21>, "error out"=w374:errorcluster)  [unwired: 11 in]
  n98 = Format Into String(w149) -> (resulting string=w138:string)  [unwired: 3 in, 1 out]
  n99 = Build Array (concatenate)(w177, w276, w261, "TrialDuration_sec", "CBVCam_Width_pix", "CBVCam_Height_pix", "CBVCam_Bit_Depth", "PupilCam_Width_pix", "PupilCam_Height_pix", "WhiskCam_Width_pix", "WhiskCam_Height_pix", "CBVCam_Exposure_Time_microsec" ("element"), "CBVCam_Binning" ("element")) -> (w168:string[])
  n100 = Format Into String(w243) -> (resulting string=w140:string)  [unwired: 3 in, 1 out]
  n101 = Multiply(x=w74, y=w76) -> (x*y=w436:dbl)
  n102 = Multiply(x="Offset (s)", y=w293) -> (x*y=w106:dbl)
  n103 = Multiply(x="Interval (s)", y=w76) -> (x*y=w314:dbl)
  n104 = Multiply(x="Duration (s)", y=w76) -> (x*y=w301:dbl)
  n105 = Multiply(x=w74, y=w34) -> (x*y=w221:dbl)
  n106 = Multiply(x=w114, y=w74) -> (x*y=w174:dbl)
  n107 = Multiply(x=w108, y=w74) -> (x*y=w113:dbl)
  n108 = call <vilib>:"IMAQ Configure Trigger3.vi"("IMAQ Session In"=w456, "Polarity"=w451, "Frame timeout (ms)"=u32 1000 ("Frame Timeout (ms)"), "Type"=w454, "Line Number"=u32 0 ("Trigger Line Number"), "Action"=w452, "error in (no error)"=w455) -> ("IMAQ Session Out"=w398:refnum<k11>, "error out"=w397:errorcluster)  [unwired: 2 in, 5 out]
  n109 = Round To Nearest(number=w301) -> (nearest integer value=w300:dbl)
  n110 = To Unsigned Long Integer(number=w174) -> (unsigned 32bit integer=w219:u32)
  n111 = To Unsigned Long Integer(number=w113) -> (unsigned 32bit integer=w109:u32)
  n112 = Round Toward -Infinity(1:w436) -> (0:w435:dbl)
  n113 = Merge Errors(w273, w272, w263) -> (w271:errorcluster)
  n114 = To Long Integer(number=w435) -> (32bit integer=w75:i32)
  n115 = flat-sequence {
    tunnel: w426 -> [w574]
    tunnel: w425 -> [w573]
    tunnel: w424 -> [w572]
    tunnel: [w572] -> w423
    tunnel: [w571] -> w421
    tunnel: [w570] -> w419
    tunnel: w417 -> [w569]
    tunnel: [w569] -> w416
    tunnel: w233 -> [w568]
    tunnel: w73 -> [w567]
    tunnel: [w566] -> w406
    tunnel: [w565] -> w404
    tunnel: [w564] -> w402
    tunnel: w232 -> [w564]
    tunnel: [w563] -> w400
    tunnel: w399 -> [w563]
    tunnel: w398 -> [w562]
    tunnel: w397 -> [w561]
    tunnel: [w560] -> w395
    tunnel: [w559] -> w393
    tunnel: w75 -> [w558]
    tunnel: [w558] -> w387
    tunnel: "Time (min)" -> [w557]
    tunnel: [w557] -> w384
    tunnel: [w556] -> w382
    tunnel: w381 -> [w556]
    tunnel: w375 -> [w555]
    tunnel: w374 -> [w554]
    tunnel: [w553] -> w373
    tunnel: [w552] -> w372
    tunnel: [w551] -> w368
    tunnel: w274 -> [w551]
    tunnel: w366 -> [w550]
    tunnel: [w550] -> w365
    tunnel: w364 -> [w549]
    tunnel: [w549] -> w363
    tunnel: w362 -> [w548]
    tunnel: [w548] -> w361
    tunnel: w360 -> [w547]
    tunnel: [w547] -> w359
    tunnel: w324 -> [w546]
    tunnel: [w546] -> w325
    tunnel: w322 -> [w545]
    tunnel: [w545] -> w323
    tunnel: w314 -> [w544]
    tunnel: [w544] -> w313
    tunnel: [w543] -> w311
    tunnel: w300 -> [w543]
    tunnel: w310 -> [w542]
    tunnel: [w542] -> w309
    tunnel: w307 -> [w541]
    tunnel: [w541] -> w306
    tunnel: [w539] -> w304
    tunnel: w221 -> [w537]
    tunnel: [w537] -> w220
    tunnel: w219 -> [w536]
    tunnel: [w536] -> w218
    tunnel: w215 -> [w535]
    tunnel: [w535] -> w214
    tunnel: [w528] -> w136
    tunnel: w118 -> [w529]
    tunnel: [w526] -> w135
    tunnel: w134 -> [w527]
    tunnel: [w534] -> w133
    tunnel: w132 -> [w534]
    tunnel: [w533] -> w131
    tunnel: w130 -> [w533]
    tunnel: [w532] -> w129
    tunnel: w128 -> [w532]
    tunnel: w117 -> [w531]
    tunnel: [w531] -> w116
    tunnel: w109 -> [w530]
    tunnel: [w530] -> w107
    tunnel: w33 -> [w525]
    tunnel: w32 -> [w524]
    tunnel: [w523] -> w31
    tunnel: [w522] -> w30
    tunnel: w5 -> [w521]
    tunnel: [w521] -> w4
    tunnel: [w625] -> w428
    tunnel: w423 -> [w624]
    tunnel: [w624] -> w422
    tunnel: w421 -> [w623]
    tunnel: [w623] -> w420
    tunnel: w419 -> [w622]
    tunnel: [w622] -> w418
    tunnel: w416 -> [w621]
    tunnel: [w621] -> w415
    tunnel: [w603] -> w412
    tunnel: [w602] -> w410
    tunnel: [w620] -> w407
    tunnel: w406 -> [w620]
    tunnel: [w619] -> w405
    tunnel: w404 -> [w619]
    tunnel: [w618] -> w403
    tunnel: w402 -> [w618]
    tunnel: [w617] -> w401
    tunnel: w400 -> [w617]
    tunnel: [w616] -> w396
    tunnel: w395 -> [w616]
    tunnel: [w615] -> w394
    tunnel: w393 -> [w615]
    tunnel: [w607] -> w391
    tunnel: [w606] -> w389
    tunnel: [w614] -> w388
    tunnel: w387 -> [w613]
    tunnel: [w613] -> w386
    tunnel: [w612] -> w385
    tunnel: w384 -> [w612]
    tunnel: [w611] -> w383
    tunnel: w382 -> [w611]
    tunnel: [w610] -> w370
    tunnel: w373 -> [w610]
    tunnel: [w609] -> w371
    tunnel: w372 -> [w609]
    tunnel: [w608] -> w28
    tunnel: w368 -> [w608]
    tunnel: w365 -> [w605]
    tunnel: w363 -> [w604]
    tunnel: w361 -> [w601]
    tunnel: w359 -> [w600]
    tunnel: w325 -> [w599]
    tunnel: w323 -> [w598]
    tunnel: [w597] -> w321
    tunnel: [w596] -> w320
    tunnel: [w595] -> w315
    tunnel: w313 -> [w595]
    tunnel: [w594] -> w312
    tunnel: w311 -> [w594]
    tunnel: w309 -> [w593]
    tunnel: [w593] -> w308
    tunnel: w306 -> [w592]
    tunnel: [w592] -> w305
    tunnel: w304 -> [w591]
    tunnel: [w591] -> w303
    tunnel: w220 -> [w590]
    tunnel: [w590] -> w29
    tunnel: w218 -> [w589]
    tunnel: [w589] -> w105
    tunnel: w214 -> [w588]
    tunnel: [w588] -> w213
    tunnel: w136 -> [w586]
    tunnel: w135 -> [w585]
    tunnel: w133 -> [w584]
    tunnel: w131 -> [w581]
    tunnel: w129 -> [w580]
    tunnel: [w578] -> w124
    tunnel: [w579] -> w123
    tunnel: [w586] -> w122
    tunnel: [w585] -> w121
    tunnel: [w584] -> w120
    tunnel: [w583] -> w115
    tunnel: w116 -> [w583]
    tunnel: [w582] -> w104
    tunnel: w107 -> [w582]
    tunnel: [w577] -> w26
    tunnel: w31 -> [w577]
    tunnel: [w576] -> w27
    tunnel: w30 -> [w576]
    tunnel: [w575] -> w3
    tunnel: w4 -> [w575]
    frame #0 {
      n116 = Initialize Array(FALSE, 3 ("dimension size")) -> (w539:bool[])
      n117 = call <vilib>:"IMAQdx Start Acquisition.vi"("error in"=w527, "Session In"=w529) -> ("error out"=w526:errorcluster, "Session Out"=w528:T2)  [unwired: 8 in]
      n118 = call <vilib>:"DAQmx Start Task.vi"("task/channels in"=w555, "error in"=w554) -> ("task out"=w553:refnum<k21>, "error out"=w552:errorcluster)  [unwired: 12 in]
      n119 = call <vilib>:"DAQmx Start Task.vi"("task/channels in"=w525, "error in"=w524) -> ("task out"=w522:refnum<k21>, "error out"=w523:errorcluster)  [unwired: 12 in]
      n120 = call <vilib>:"IMAQdx Configure Grab.vi"("error in"=w574, "Session In"=w573) -> ("error out"=w570:errorcluster, "Session Out"=w571:T2)  [unwired: 8 in]
      n121 = call <vilib>:"IMAQ Start.vi"("error in (no error)"=w561, "IMAQ Session In"=w562) -> ("error out"=w559:errorcluster, "IMAQ Session Out"=w560:refnum<k11>)  [unwired: 8 out]
      n122 = call <vilib>:"IMAQdx Start Acquisition.vi"("error in"=w567, "Session In"=w568) -> ("error out"=w565:errorcluster, "Session Out"=w566:T2)  [unwired: 8 in]
    }
    frame #1 {
      n123 = local write "CBV Camera"(FALSE ("Finished Acquiring")) -> ()
      n124 = call <vilib>:"DAQmx Start Task.vi"("task/channels in"=w581, "error in"=w580) -> ("task out"=w578:refnum<k21>, "error out"=w579:errorcluster)  [unwired: 12 in]
      n125 = Tick Count (ms)() -> (millisecond timer value=w625:u32)
      n126 = call <vilib>:"DAQmx Start Task.vi"("task/channels in"=w605, "error in"=w604) -> ("task out"=w607:refnum<k21>, "error out"=w606:errorcluster)  [unwired: 12 in]
      n127 = call <vilib>:"DAQmx Start Task.vi"("task/channels in"=w601, "error in"=w600) -> ("task out"=w603:refnum<k21>, "error out"=w602:errorcluster)  [unwired: 12 in]
      n128 = Tick Count (ms)() -> (millisecond timer value=w614:u32)
      n129 = call <vilib>:"DAQmx Start Task.vi"("task/channels in"=w599, "error in"=w598) -> ("task out"=w597:refnum<k21>, "error out"=w596:errorcluster)  [unwired: 12 in]
    }
  }
  n130 = Cluster To Array(cluster="Notes:") -> (array=w283:string[])
  n131 = TDMS Open(6:FALSE ("disable buffering? (T)"), 7:enum16{"1.0", "2.0"}."1.0" ("file format version (2.0)"), 8:w271, 10:T5."create" ("operation (0:open)"), 11:w282) -> (0:w277:errorcluster, 3:w278:refnum<k34>)  [unwired: 2 in]
  n132 = Build Array(w112, w111, w110, w51, w50, w247, w239, w173, w238, w137, w138, w139, w140, "Exposure Time (microsec)", w142) -> (w258:string[])
  n133 = Build Array (concatenate)(w283, w258) -> (w275:string[])
  n134 = TDMS Set Properties(5:w275, 7:w168, 8:w277, 11:w278) -> (0:w270:errorcluster, 3:w274:refnum<k34>)  [unwired: 2 in, 2 out]
  n135 = call <vilib>:"Simple Error Handler.vi"("error source (\" \")"="Error in creating .tdms notes" ("error source (\" \")"), "error in (no error)"=w270) -> ()  [unwired: 3 in, 5 out]
  n136 = call-poly <vilib>:"DAQmx Write.vi"("task/channels in"=w212, "data"=TRUE, "error in"=w213) -> ("task out"=w210:refnum<k21>, "error out"=w208:errorcluster)  [unwired: 10 in, 1 out]
  n137 = TDMS Open(6:FALSE ("disable buffering? (T)"), 7:enum16{"1.0", "2.0"}."1.0" ("file format version (2.0)"), 10:T5."create" ("operation (0:open)"), 11:w2) -> (3:w5:refnum<k34>)  [unwired: 3 in, 1 out]
  n138 = while {
    tunnel: w26 -> [w648]
    tunnel: w27 -> [w647]
    tunnel: [w646] -> w12
    tunnel: [w634] -> w13
    tunnel: [w645] -> w23
    shift-right: [w638] -> _
    shift-left: _ -> [w629]
    tunnel: [w634] -> w22
    tunnel: w29 -> [w632]
    tunnel: w3 -> [w626]
    i -> [w630]
    stop <- w635 stop-if-true
    n139 = To Long Integer(number=w632) -> (32bit integer=w633:i32)
    n140 = call-poly <vilib>:"DAQmx Read.vi"("task/channels in"=w647, "error in"=w648) -> ("task out"=w645:refnum<k21>, "data"=w643:waveform(dbl)[], "error out"=w637:errorcluster)  [unwired: 11 in]
    n141 = Greater?(x=w629, y=w630) -> (0:→"Dev2 Analog":bool)
    n142 = TDMS Write(0:w626, 5:"Analog Data" ("group name in (Untitled)"), 9:w643, 11:w637) -> (4:w646:refnum<k34>, 15:w634:errorcluster)  [unwired: 2 in, 2 out]
    n143 = Index Array(array=w643, index=0) -> (element=w641:waveform(dbl))
    n144 = Unbundle By Name(w641) -> ("Y"=w640:dbl[])
    n145 = local read "CBV Camera"() -> (w628:bool)
    n146 = local read "stop"() -> (w627:bool)
    n147 = Array Size(array=w640) -> (size(s)=w639:i32)
    n148 = Add(x=w639, y=w629) -> (x+y=w638:i32)
    "Dev2 Analog Samples" <- w638
    n149 = Greater Or Equal?(x=w638, y=w633) -> (x >= y?=w636:bool)
    n150 = Compound Arithmetic op=OR(w634, w636, w627, w628) -> (w635:bool)
  }
  n151 = while {
    tunnel: w396 -> [w694]
    tunnel: w394 -> [w695]
    tunnel: [w659] -> w440
    tunnel: [w657] -> w441
    tunnel: [w689] -> w439
    tunnel: [w684] -> w392
    tunnel: w391 -> [w684]
    tunnel: [w683] -> w390
    tunnel: w389 -> [w683]
    tunnel: w388 -> [w682]
    tunnel: w386 -> [w681]
    tunnel: w385 -> [w680]
    tunnel: w383 -> [w656]
    tunnel: w321 -> [w677]
    tunnel: w320 -> [w676]
    tunnel: [w675] -> w319
    tunnel: [w674] -> w318
    tunnel: w315 -> [w669]
    tunnel: w312 -> [w668]
    tunnel: w308 -> [w666]
    tunnel: w305 -> [w664]
    tunnel: w303 -> [w673]
    tunnel: w106 -> [w667]
    tunnel: w254 -> [w671]
    tunnel: w210 -> [w661]
    tunnel: [w661] -> w209
    tunnel: [w660] -> w207
    tunnel: w208 -> [w660]
    tunnel: w72 -> [w651]
    i -> [w652]
    stop <- w662 stop-if-true
    # "Track ISI"
    n152 = Tick Count (ms)() -> (millisecond timer value=w687:u32)
    n153 = Greater?(x=w652, y=w651) -> (0:→"CBV Cam":bool)
    n154 = call <vilib>:"IMAQ Extract Buffer.vi"("error in (no error)"=w695, "Buffer to extract"=w652, "IMAQ Session In"=w694) -> ("error out"=w688:errorcluster, "Buffer Number"=w670:i32, "Image Out"=w649:T1, "IMAQ Session Out"=w657:refnum<k11>)  [unwired: 5 out]
    "Last CBV\nBuffer" <- w670
    "?" <- w649
    n155 = case shown="True" w671 {
      selector: w671 -> [w697 _]
      tunnel: w670 -> [_ w707]
      tunnel: w669 -> [_ w706]
      tunnel: w668 -> [_ w705]
      tunnel: w667 -> [_ w704]
      tunnel: w666 -> [_ w701]
      tunnel: [0.0 ("element") w698] -> w665
      tunnel: w664 -> [_ w700]
      tunnel: [w697 w699] -> w663
      frame False {
      }
      frame True {
        n156 = Quotient & Remainder(x=w707, y=w706) -> (x-y*floor(x/y)=w709:dbl, floor(x/y)=w702:dbl)
        n157 = Add(x=w705, y=w704) -> (x+y=w708:dbl)
        n158 = Quotient & Remainder(x=w702, y=w701) -> (x-y*floor(x/y)=w703:dbl)  [unwired: 1 out]
        n159 = In Range and Coerce(upper limit=w708, x=w709, lower limit=w704) -> (In Range?=w699:bool)  [unwired: 1 out]
        n160 = Index Array(array=w700, index=w703) -> (element=w698:dbl)
      }
    }
    n161 = Subtract(x=w687, y=w682) -> (x-y=w686:u32)
    n162 = call <vilib>:"Calculate Frames per Second.vi"("Update Interval (ms)"=u32 2000, "Buffer Number"=w670) -> ("Processed Frames/s"=→"CBV Cam":dbl)  [unwired: 7 in, 2 out]
    n163 = Multiply(x=w686, y=1.667e-05) -> (x*y=w685:dbl)
    n164 = Greater Or Equal?(x=w670, y=w681) -> (x >= y?=w655:bool)
    n165 = call "IMAQ ImageToArray"("error in (no error)"=w688, "Image"=w649) -> ("error out"=w693:errorcluster, "Image Pixels (I16)"=w692:i16[][])  [unwired: 2 in, 3 out]
    n166 = Bundle("Time (min)"=w680, w685) -> (→"Time Elapsed (Min)":cluster{"Time (min)":dbl, dbl})  [unwired: 1 in]
    n167 = local write "stop"("stop") -> ()
    n168 = Replace Array Subset(array=w673, new element=w663, index=w665) -> (w672:bool[])
    "Solenoids" <- w672
    n169 = call-poly <vilib>:"DAQmx Write.vi"("task/channels in"=w677, "data"=w672, "error in"=w676) -> ("task out"=w675:refnum<k21>, "error out"=w674:errorcluster)  [unwired: 10 in, 1 out]
    n170 = Write to Binary File(file (use dialog)=w656, data=w692, error in=w693, 5:FALSE ("prepend array or string size? (T)"), 9:T11."big-endian, network order" ("byte order (0:big-endian, network order)")) -> (refnum out=w689:refnum<file>, error out=w659:errorcluster)  [unwired: 1 in, 1 out]
    n171 = Compound Arithmetic op=OR(w659, w655, "stop") -> (w662:bool)
    "CBV Camera" <- w662
  }
  n172 = while {
    tunnel: w124 -> [w736]
    tunnel: [w737] -> w89
    tunnel: w123 -> [w737]
    tunnel: [w736] -> w88
    tunnel: [w725] -> w86
    tunnel: [w726] -> w87
    tunnel: [w735] -> w85
    tunnel: w122 -> [w734]
    tunnel: w121 -> [w733]
    tunnel: w115 -> [w732]
    tunnel: w120 -> [w731]
    shift-right: [w724] -> _
    shift-left: _ -> [w730]
    shift-right: [w729] -> _
    shift-left: u32 0 ("New Lost") -> [w723]
    shift-right: [w728] -> w83
    shift-left: u32[] [] ("NewBuffNum") -> [w717]
    shift-right: [w727] -> w84
    shift-left: u32[] [] ("NewNumLost") -> [w718]
    tunnel: w104 -> [w716]
    tunnel: w72 -> [w713]
    i -> [w714]
    stop <- w719 stop-if-true
    n173 = call <vilib>:"IMAQdx Get Image.vi"("Buffer Number Mode (Next)"=IMAQdx_Buffer_Number_Mode."Next", "error in"=w733, "Image In"=w732, "Session In"=w734) -> ("error out"=w744:errorcluster, "Buffer Number Out"=w724:u32, "Image Out"=w710:T1, "Session Out"=w725:T2)  [unwired: 4 in]
    "Last Whisk\nBuffer 2" <- w724
    "?" <- w710
    n174 = Greater?(x=w714, y=w713) -> (0:→"Pupil Cam":bool)
    n175 = call "TrackPupilDroppedFrames_IOS.vi"("NumLost"=w718, "BuffNum"=w717, "Curr Buffer"=w724, "Prev Lost"=w723, "Prev Buffer"=w730) -> ("New Lost"=w729:u32, "NewNumLost"=w727:u32[], "NewBuffNum"=w728:u32[])  [unwired: 4 in]
    "Dropped 2" <- w729
    n176 = call "IMAQ ImageToArray"("error in (no error)"=w744, "Image"=w710) -> ("error out"=w743:errorcluster, "Image Pixels (U8)"=w742:u8[][])  [unwired: 2 in, 3 out]
    n177 = Add(x=w724, y=w723) -> (x+y=w722:u32)
    n178 = Greater Or Equal?(x=w722, y=w716) -> (x >= y?=w720:bool)
    n179 = Write to Binary File(file (use dialog)=w731, data=w742, error in=w743, 5:FALSE ("prepend array or string size? (T)"), 9:T11."little-endian" ("byte order (0:big-endian, network order)")) -> (refnum out=w735:refnum<file>, error out=w726:errorcluster)  [unwired: 1 in, 1 out]
    n180 = local read "stop"() -> (w712:bool)
    n181 = local read "CBV Camera"() -> (w711:bool)
    n182 = call <vilib>:"Calculate Frames per Second.vi"("Update Interval (ms)"=u32 2000, "Buffer Number"=w724) -> ("Processed Frames/s"=→"Pupil Cam Fs":dbl)  [unwired: 7 in, 2 out]
    n183 = Unbundle By Name(w726) -> ("status"=w721:bool)
    n184 = Compound Arithmetic op=OR(w721, w720, w712, w711) -> (w719:bool)
  }
  n185 = while {
    tunnel: w412 -> [w773]
    tunnel: [w774] -> w411
    tunnel: w410 -> [w774]
    tunnel: [w773] -> w409
    tunnel: [w766] -> w230
    tunnel: [w767] -> w294
    tunnel: [w772] -> w408
    tunnel: w407 -> [w771]
    tunnel: w405 -> [w770]
    tunnel: w403 -> [w769]
    tunnel: w401 -> [w768]
    shift-right: [w754] -> _
    shift-left: _ -> [w752]
    shift-right: [w749] -> _
    shift-left: u32 0 ("New Lost") -> [w753]
    shift-right: [w750] -> w222
    shift-left: u32[] [] ("NewBuffNum") -> [w751]
    shift-right: [w756] -> w353
    shift-left: u32[] [] ("NewNumLost") -> [w755]
    tunnel: w105 -> [w764]
    tunnel: w72 -> [w757]
    i -> [w758]
    stop <- w761 stop-if-true
    n186 = call <vilib>:"IMAQdx Get Image.vi"("Buffer Number Mode (Next)"=IMAQdx_Buffer_Number_Mode."Next", "error in"=w770, "Image In"=w769, "Session In"=w771) -> ("error out"=w780:errorcluster, "Buffer Number Out"=w754:u32, "Image Out"=w746:T1, "Session Out"=w766:T2)  [unwired: 4 in]
    "Last Whisk\nBuffer" <- w754
    "?" <- w746
    n187 = Greater?(x=w758, y=w757) -> (0:→"Whisk Cam":bool)
    n188 = call "IMAQ ImageToArray"("error in (no error)"=w780, "Image"=w746) -> ("error out"=w779:errorcluster, "Image Pixels (U8)"=w778:u8[][])  [unwired: 2 in, 3 out]
    n189 = call "TrackWhiskDroppedFrames_IOS.vi"("NumLost"=w755, "BuffNum"=w751, "Curr Buffer"=w754, "Prev Lost"=w753, "Prev Buffer"=w752) -> ("New Lost"=w749:u32, "NewNumLost"=w756:u32[], "NewBuffNum"=w750:u32[])  [unwired: 4 in]
    "Dropped" <- w749
    n190 = Add(x=w754, y=w753) -> (x+y=w765:u32)
    n191 = Greater Or Equal?(x=w765, y=w764) -> (x >= y?=w762:bool)
    n192 = Write to Binary File(file (use dialog)=w768, data=w778, error in=w779, 5:FALSE ("prepend array or string size? (T)"), 9:T11."little-endian" ("byte order (0:big-endian, network order)")) -> (refnum out=w772:refnum<file>, error out=w767:errorcluster)  [unwired: 1 in, 1 out]
    n193 = local read "stop"() -> (w748:bool)
    n194 = local read "CBV Camera"() -> (w747:bool)
    n195 = call <vilib>:"Calculate Frames per Second.vi"("Update Interval (ms)"=u32 2000, "Buffer Number"=w754) -> ("Processed Frames/s"=→"Whisk Cam Fs":dbl)  [unwired: 7 in, 2 out]
    n196 = Unbundle By Name(w767) -> ("status"=w763:bool)
    n197 = Compound Arithmetic op=OR(w763, w762, w748, w747) -> (w761:bool)
  }
  n198 = while {
    tunnel: w428 -> [w798]
    tunnel: w422 -> [w796]
    tunnel: w420 -> [w795]
    tunnel: w418 -> [w794]
    tunnel: w415 -> [w792]
    tunnel: [w793] -> w119
    tunnel: [w784] -> w413
    tunnel: [w792] -> w414
    tunnel: w72 -> [w787]
    i -> [w788]
    stop <- w785 stop-if-true
    n199 = Tick Count (ms)() -> (millisecond timer value=w800:u32)
    n200 = Subtract(x=w800, y=w798) -> (x-y=w801:u32)
    n201 = Divide(x=w801, y=u32 1000) -> (x/y=w797:dbl)
    n202 = Greater?(x=w788, y=w787) -> (0:→"Web Cam":bool)
    n203 = call "GrabWebCam_IOS.vi"("Session In"=w795, "Image In"=w796, "Trial Time"=w797, "AVI Refnum"=w792, "error in"=w794) -> ("Session Out"=w793:T2, "WebCam Img Out"=→"?":T1, "Buffer Number Out"=w791:u32, "error out"=w784:errorcluster)  [unwired: 7 in]
    n204 = local read "CBV Camera"() -> (w786:bool)
    n205 = local read "stop"() -> (w783:bool)
    n206 = call <vilib>:"Calculate Frames per Second.vi"("Update Interval (ms)"=u32 5000, "Buffer Number"=w791) -> ("Processed Frames/s"=→"Web Cam Fs":dbl)  [unwired: 7 in, 2 out]
    n207 = Compound Arithmetic op=OR(w784, w783, w786) -> (w785:bool)
  }
  n208 = while {
    tunnel: w371 -> [w825]
    tunnel: w370 -> [w824]
    tunnel: w28 -> [w823]
    tunnel: [w822] -> w78
    tunnel: [w810] -> w77
    tunnel: [w821] -> w367
    shift-right: [w814] -> _
    shift-left: w72 -> [w805]
    tunnel: [w810] -> w169
    tunnel: w29 -> [w808]
    i -> [w806]
    stop <- w811 stop-if-true
    n209 = To Long Integer(number=w808) -> (32bit integer=w809:i32)
    n210 = call-poly <vilib>:"DAQmx Read.vi"("task/channels in"=w824, "error in"=w825) -> ("task out"=w821:refnum<k21>, "data"=w819:waveform(dbl)[], "error out"=w813:errorcluster)  [unwired: 11 in]
    n211 = Greater?(x=w805, y=w806) -> (0:→"Dev1 Analog":bool)
    n212 = TDMS Write(0:w823, 5:"Analog Data" ("group name in (Untitled)"), 9:w819, 11:w813) -> (4:w822:refnum<k34>, 15:w810:errorcluster)  [unwired: 2 in, 2 out]
    n213 = Index Array(array=w819, index=0) -> (element=w817:waveform(dbl))
    n214 = Unbundle By Name(w817) -> ("Y"=w816:dbl[])
    n215 = local read "CBV Camera"() -> (w804:bool)
    n216 = local read "stop"() -> (w803:bool)
    n217 = Array Size(array=w816) -> (size(s)=w815:i32)
    n218 = Add(x=w815, y=w805) -> (x+y=w814:i32)
    "Dev1 Analog Samples" <- w814
    n219 = Greater Or Equal?(x=w814, y=w809) -> (x >= y?=w812:bool)
    n220 = Compound Arithmetic op=OR(w810, w812, w803, w804) -> (w811:bool)
  }
  n221 = call <vilib>:"DAQmx Stop Task.vi"("task/channels in"=w23, "error in"=w22) -> ("task out"=w25:refnum<k21>, "error out"=w24:errorcluster)  [unwired: 12 in]
  n222 = call <vilib>:"DAQmx Stop Task.vi"("task/channels in"=w367, "error in"=w169) -> ("task out"=w296:refnum<k21>, "error out"=w295:errorcluster)  [unwired: 12 in]
  n223 = call <vilib>:"IMAQ Extract Buffer.vi"("error in (no error)"=w440, "Buffer to extract"=-1, "IMAQ Session In"=w441) -> ("error out"=w462:errorcluster, "IMAQ Session Out"=w461:refnum<k11>)  [unwired: 7 out]
  n224 = Close File(refnum=w439, error in=w77) -> (path=w347:path)  [unwired: 1 out]
  n225 = Delete From Array(array=w222, length=1, index=0) -> (array with subset deleted=w182:u32[])  [unwired: 1 out]
  n226 = call-poly <vilib>:"DAQmx Write.vi"("task/channels in"=w209, "data"=FALSE, "error in"=w207) -> ("task out"=w206:refnum<k21>, "error out"=w204:errorcluster)  [unwired: 10 in, 1 out]
  n227 = Delete From Array(array=w353, length=1, index=0) -> (array with subset deleted=w183:u32[])  [unwired: 1 out]
  n228 = call <vilib>:"DAQmx Stop Task.vi"("task/channels in"=w88, "error in"=w89) -> ("task out"=w61:refnum<k21>, "error out"=w62:errorcluster)  [unwired: 12 in]
  n229 = call <vilib>:"DAQmx Stop Task.vi"("task/channels in"=w409, "error in"=w411) -> ("task out"=w59:refnum<k21>, "error out"=w60:errorcluster)  [unwired: 12 in]
  n230 = Delete From Array(array=w84, length=1, index=0) -> (array with subset deleted=w91:u32[])  [unwired: 1 out]
  n231 = Delete From Array(array=w83, length=1, index=0) -> (array with subset deleted=w90:u32[])  [unwired: 1 out]
  n232 = call <vilib>:"IMAQdx Close Camera.vi"("error in"=w294, "Session In"=w230) -> ()  [unwired: 9 in, 1 out]
  n233 = Close File(refnum=w408, error in=w294) -> (path=w345:path, error out=w344:errorcluster)
  n234 = call "IMAQ AVI2 Close"("error in (no error)"=w413, "AVI Refnum"=w414) -> ("error out"=w346:errorcluster)  [unwired: 9 in]
  n235 = call <vilib>:"IMAQdx Close Camera.vi"("error in"=w413, "Session In"=w119) -> ()  [unwired: 9 in, 1 out]
  n236 = call <vilib>:"DAQmx Clear Task.vi"("task in"=w25, "error in"=w24) -> ()  [unwired: 13 in, 1 out]
  n237 = call <vilib>:"IMAQdx Close Camera.vi"("error in"=w87, "Session In"=w86) -> ()  [unwired: 9 in, 1 out]
  n238 = Close File(refnum=w85, error in=w87) -> (path=w80:path, error out=w79:errorcluster)
  n239 = Build Array(w182, w183) -> (w185:u32[][])
  n240 = call <vilib>:"DAQmx Clear Task.vi"("task in"=w296, "error in"=w295) -> ()  [unwired: 13 in, 1 out]
  n241 = call <vilib>:"DAQmx Stop Task.vi"("task/channels in"=w206, "error in"=w204) -> ("task out"=w205:refnum<k21>, "error out"=w203:errorcluster)  [unwired: 12 in]
  n242 = call <vilib>:"DAQmx Stop Task.vi"("task/channels in"=w319, "error in"=w318) -> ("task out"=w317:refnum<k21>, "error out"=w316:errorcluster)  [unwired: 12 in]
  n243 = call <vilib>:"DAQmx Stop Task.vi"("task/channels in"=w392, "error in"=w390) -> ("task out"=w63:refnum<k21>, "error out"=w64:errorcluster)  [unwired: 12 in]
  n244 = call <vilib>:"IMAQ Close.vi"("error in (no error)"=w462, "IMAQ Session In"=w461) -> ("error out"=w463:errorcluster)  [unwired: 9 out]
  n245 = Build Array(w90, w91) -> (w93:u32[][])
  n246 = call <vilib>:"DAQmx Clear Task.vi"("task in"=w59, "error in"=w60) -> ()  [unwired: 13 in, 1 out]
  n247 = call <vilib>:"DAQmx Clear Task.vi"("task in"=w61, "error in"=w62) -> ()  [unwired: 13 in, 1 out]
  n248 = Array To Spreadsheet String(delimiter (Tab)=",", array=w183, 3:"%d" ("format string")) -> (spreadsheet string=w223:string)
  n249 = Transpose 2D Array(2D array=w185) -> (transposed array=w184:u32[][])
  n250 = Array To Spreadsheet String(delimiter (Tab)=",", array=w182, 3:"%d" ("format string")) -> (spreadsheet string=w224:string)
  n251 = Move(source path=w80, error in=w79, 10:"Target Path") -> (error out=w81:errorcluster)  [unwired: 2 in, 2 out]
  n252 = Move(source path=w345, error in=w344, 10:"Target Path") -> (error out=w342:errorcluster)  [unwired: 2 in, 2 out]
  n253 = Array To Spreadsheet String(delimiter (Tab)=",", array=w91, 3:"%d" ("format string")) -> (spreadsheet string=w94:string)
  n254 = Transpose 2D Array(2D array=w93) -> (transposed array=w92:u32[][])
  n255 = Array To Spreadsheet String(delimiter (Tab)=",", array=w90, 3:"%d" ("format string")) -> (spreadsheet string=w95:string)
  n256 = Move(source path=w171, error in=w346, 10:"Target Path") -> (error out=w341:errorcluster)  [unwired: 2 in, 2 out]
  n257 = call <vilib>:"DAQmx Clear Task.vi"("task in"=w63, "error in"=w64) -> ()  [unwired: 13 in, 1 out]
  n258 = TDMS Close(8:w13, 11:w12) -> (0:w21:errorcluster, 3:w1:path)
  n259 = call <vilib>:"DAQmx Clear Task.vi"("task in"=w205, "error in"=w203) -> ()  [unwired: 13 in, 1 out]
  n260 = for {
    N: w172 -> [_]
    tunnel: w457 -> [w829] mode=indexing
    shift-right: [w827] -> w349
    shift-left: w463 -> [w828]
    n261 = call "IMAQ Dispose"("All Images? (No)"=FALSE, "Image"=w829, "error in (no error)"=w828) -> ("error out"=w827:errorcluster)  [unwired: 3 out]
  }
  n262 = call <vilib>:"DAQmx Clear Task.vi"("task in"=w317, "error in"=w316) -> ()  [unwired: 13 in, 1 out]
  n263 = call <vilib>:"Trim Whitespace.vi"("string"=w224) -> ("trimmed string"=w54:string)  [unwired: 1 in]
  n264 = call <vilib>:"Trim Whitespace.vi"("string"=w223) -> ("trimmed string"=w53:string)  [unwired: 1 in]
  n265 = Number To Decimal String(number=w184) -> ()  [unwired: 1 in, 1 out]
  n266 = call <vilib>:"Trim Whitespace.vi"("string"=w95) -> ("trimmed string"=w55:string)  [unwired: 1 in]
  n267 = call <vilib>:"Trim Whitespace.vi"("string"=w94) -> ("trimmed string"=w56:string)  [unwired: 1 in]
  n268 = Number To Decimal String(number=w92) -> ()  [unwired: 1 in, 1 out]
  n269 = call <vilib>:"Simple Error Handler.vi"("error in (no error)"=w81) -> ()  [unwired: 1 in, 8 out]
  n270 = call <vilib>:"Simple Error Handler.vi"("error in (no error)"=w342) -> ()  [unwired: 1 in, 8 out]
  n271 = Path To String(path=w1) -> (string=w19:string)
  n272 = call <vilib>:"Simple Error Handler.vi"("error in (no error)"=w341) -> ()  [unwired: 1 in, 8 out]
  n273 = TDMS Defragment(4:w21, 7:w1) -> (0:w15:errorcluster)
  n274 = Build Array(w55, w56, w54, w53) -> (w52:string[])
  n275 = Concatenate Strings(w19, "_index" ("string")) -> (w17:string)
  n276 = Move(source path=w347, error in=w349, 10:"Target Path") -> (error out=w348:errorcluster)  [unwired: 2 in, 2 out]
  n277 = String To Path(string=w17) -> (path=w16:path)
  n278 = call <vilib>:"Simple Error Handler.vi"("error in (no error)"=w348) -> ()  [unwired: 1 in, 8 out]
  n279 = Move(source path=w1, error in=w15, 10:"Target Path") -> (error out=w20:errorcluster)  [unwired: 2 in, 2 out]
  n280 = Move(source path=w16, error in=w15, 10:"Target Path") -> (error out=w14:errorcluster)  [unwired: 2 in, 2 out]
  n281 = TDMS Set Properties(5:w52, 7:string[] ["PupilCam_DroppedFrameIndex", "PupilCam_NumberDropped", "WhiskCam_DroppedFrameIndex", "WhiskCam_NumberDropped"] ("channel name(s) in (Untitled)"), 8:w77, 11:w78) -> (0:w231:errorcluster, 3:w229:refnum<k34>)  [unwired: 2 in, 2 out]
  n282 = call <vilib>:"Simple Error Handler.vi"("error in (no error)"=w20) -> ()  [unwired: 1 in, 8 out]
  n283 = call <vilib>:"Simple Error Handler.vi"("error in (no error)"=w14) -> ()  [unwired: 1 in, 8 out]
  n284 = TDMS Close(8:w231, 11:w229) -> (0:w350:errorcluster, 3:w338:path)
  n285 = Path To String(path=w338) -> (string=w340:string)
  n286 = TDMS Defragment(4:w350, 7:w338) -> (0:w335:errorcluster)
  n287 = Concatenate Strings(w340, "_index" ("string")) -> (w337:string)
  n288 = String To Path(string=w337) -> (path=w336:path)
  n289 = Move(source path=w338, error in=w335, 10:"Target Path") -> (error out=w343:errorcluster)  [unwired: 2 in, 2 out]
  n290 = Move(source path=w336, error in=w335, 10:"Target Path") -> (error out=w82:errorcluster)  [unwired: 2 in, 2 out]
  n291 = call <vilib>:"Simple Error Handler.vi"("error in (no error)"=w343) -> ()  [unwired: 1 in, 8 out]
  n292 = call <vilib>:"Simple Error Handler.vi"("error in (no error)"=w82) -> ()  [unwired: 1 in, 8 out]
